vi "Do Process.vi"(8 "error in (no error)":errorcluster, 11 "Template Service in":refnum<class "Sequencer.lvclass">) -> (0 "error out":errorcluster, 3 "Template Service out":refnum<class "Sequencer.lvclass">)   [LabVIEW 2024, in "Ramses Sequencer.lvlib" / "Sequencer.lvclass"]
uses:
  Sequencer.lvclass
  typedef/Sequencer State -- enum.ctl
  Sequence/Sequence.lvclass
  Base Step/Base Step.lvclass
  Program Files (x86)/Enterative/Ramses Framework/Ramses Framework.lvlibp/Service/Service.lvclass
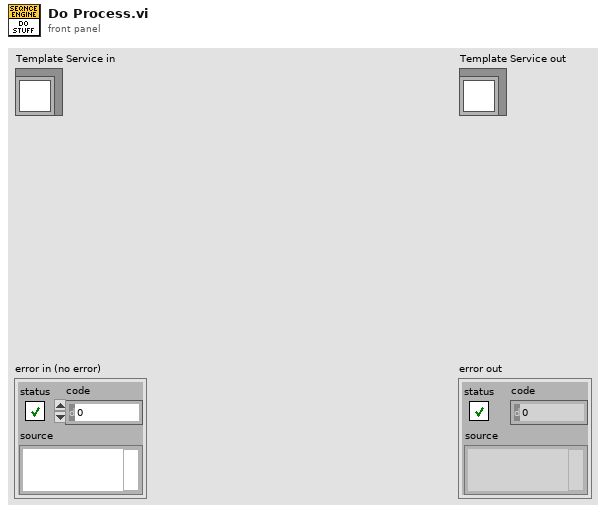
[diagram p1: front panel]
types:
  T1 = typedef "Ramses Sequencer.lvlib/Sequencer.lvclass/Sequencer State -- enum.ctl" = enum16{"Idle", "Running", "Paused", "Complete"}
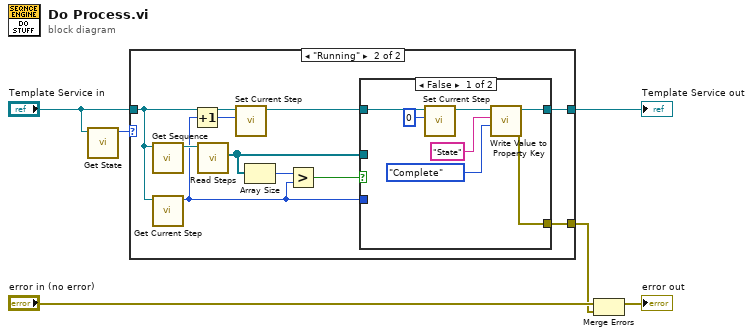
[diagram p0: block diagram]
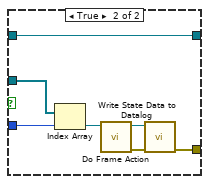
[diagram p3: hidden frame]
diagram:
  n1 = call "Get State.vi"("Sequencer in"="Template Service in") -> ("Sequencer State"=w1:T1)  [unwired: 9 in, 1 out]
  n2 = case shown="\"Running\"" w1 {
    tunnel: "Template Service in" -> [w7 w10]
    tunnel: [w7 w14] -> w5
    tunnel: [_ w16] -> w3
    frame Default {
    }
    frame "Running" {
      n3 = call "Get Sequence.vi"("Sequencer in"=w10) -> ("Sequence"=w17:refnum<class "Sequence.lvclass">)  [unwired: 9 in, 1 out]
      n4 = call "Get Current Step.vi"("Sequencer in"=w10) -> ("Current Step"=w13:u32)  [unwired: 9 in, 1 out]
      n5 = Increment(x=w13) -> (x+1=w8:u32)
      n6 = call-dynamic "Read Steps.vi"("Sequence in"=w17) -> ("Steps"=w15:refnum<class "Base Step.lvclass">[])  [unwired: 8 in, 2 out]
      n7 = call "Set Current Step.vi"("Current Step"=w8, "Sequencer in"=w10) -> ("Sequencer out"=w9:refnum<class "Sequencer.lvclass">)  [unwired: 8 in, 1 out]
      n8 = Array Size(array=w15) -> (size(s)=w11:i32)
      n9 = Greater?(x=w11, y=w13) -> (0:w12:bool)
      n10 = case shown="False" w12 {
        tunnel: w13 -> [_ w31]
        tunnel: [w18 w27] -> w16
        tunnel: w15 -> [_ w30]
        tunnel: w9 -> [w24 w29]
        tunnel: [w21 w29] -> w14
        frame False {
          n11 = call "Set Current Step.vi"("Current Step"=u32 0, "Sequencer in"=w24) -> ("Sequencer out"=w22:refnum<class "Sequencer.lvclass">)  [unwired: 8 in, 1 out]
          n12 = call "Write Value to Property Key.vi"("Value"=Sequencer_State_--_enum."Complete" ("Sequencer State"), "Key"="State", "Service in"=w22) -> ("error out"=w18:errorcluster, "Service out"=w21:refnum<class "Sequencer.lvclass">)  [unwired: 7 in]
        }
        frame True {
          n13 = Index Array(array=w30, index=w31) -> (element=w25:refnum<class "Base Step.lvclass">)
          n14 = call-dynamic "Do Frame Action.vi"("Base Step in"=w25) -> ("error out"=w26:errorcluster, "Base Step out"=w28:refnum<class "Base Step.lvclass">)  [unwired: 9 in]
          n15 = call "Write State Data to Datalog.vi"("error in (no error)"=w26, "Base Step in"=w28) -> ("error out"=w27:errorcluster)  [unwired: 9 in]
        }
      }
    }
  }
  "Template Service out" <- w5
  n16 = Merge Errors("error in (no error)", w3) -> (→"error out":errorcluster)
